vi "Timeout.vi"(8 "error in (no error)":errorcluster, 10 "allow send timeout":bool=TRUE, 11 "BaseDriver in":refnum<class "BaseDriver.lvclass">) -> (0 "error out":errorcluster, 2 "timed out?":bool, 3 "BaseDriver out":refnum<class "BaseDriver.lvclass">)   [LabVIEW 2013, in "BaseDriver.lvclass"]
doc: "Handles a timeout that occurs when an expected response to a message doesn't arrive on time. Tries to resend the message a fixed number of times"
uses:
  BaseDriver.lvclass
  BaseDriver.lvclass/BaseDriver.ctl
  Message/BaseMessage/BaseMessage.lvclass
  driver_state.ctl
  Responder/BaseResponder/BaseResponder.lvclass
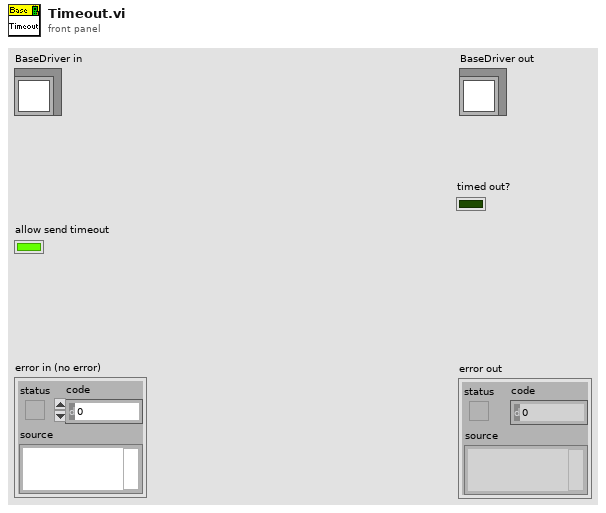
[diagram p1: front panel]
types:
  T1 = typedef "driver_state.ctl" = enum16{"Idle", "Wait for ack"}
  T2 = typedef "response.ctl" = cluster{"driver status":T3, "Sender":string, "Type":i32, "Variant":variant}
  T3 = typedef "driver_status.ctl" = enum16{"Normal", "Startup", "Connection lost", "Reconnected", "Timeout", "Idle", "Busy"}
  T4 = typedef "message_queue.ctl" = refnum<queue>
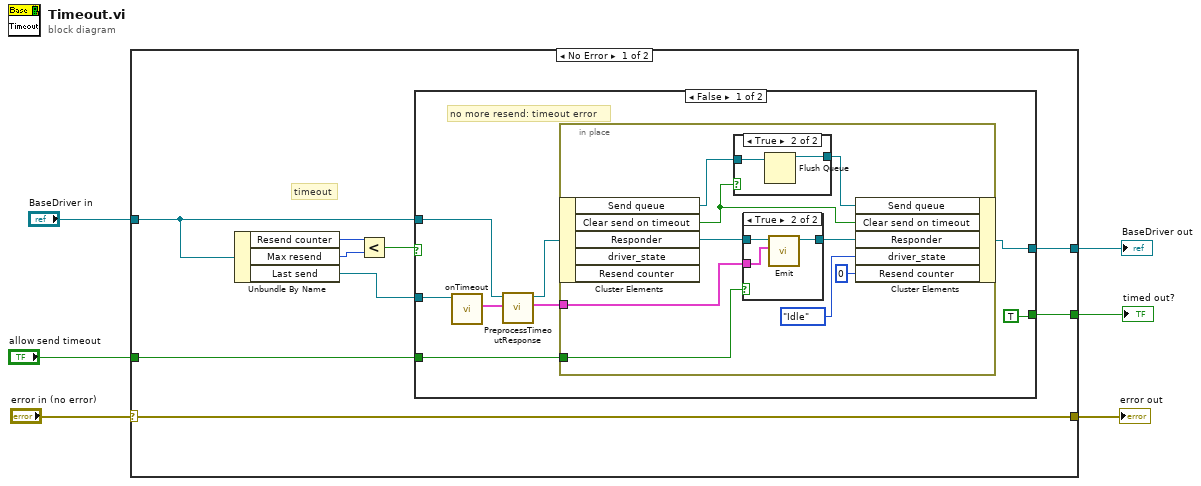
[diagram p0: block diagram]
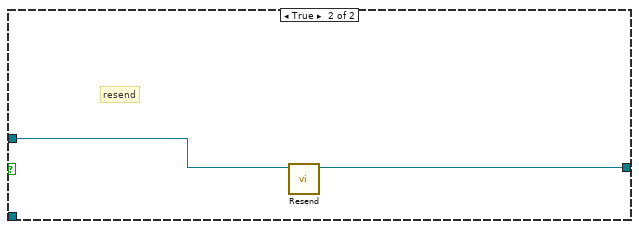
[diagram p4: hidden frame]
diagram:
  n1 = case shown="No Error" "error in (no error)" {
    selector: "error in (no error)" -> [w10 w42]
    tunnel: "BaseDriver in" -> [w12 w43]
    tunnel: [w11 w43] -> w5
    tunnel: [w10 w42] -> w3
    tunnel: [w8 _] -> w2
    tunnel: "allow send timeout" -> [w7 _]
    frame No Error {
      # "timeout"
      n2 = Unbundle By Name(w12) -> ("Resend counter"=w15:i32, "Max resend"=w14:i32, "Last send"=w9:refnum<class "BaseMessage.lvclass">)
      n3 = Less?(x=w15, y=w14) -> (x < y?=w13:bool)
      n4 = case shown="False" w13 {
        tunnel: w12 -> [w19 w41]
        tunnel: [w20 w40] -> w11
        tunnel: w9 -> [w23 _]
        tunnel: [TRUE _] -> w8
        tunnel: w7 -> [w21 _]
        frame False {
          # "no more resend: timeout error"
          n5 = call-dynamic "onTimeout.vi"("Last sent message in"=w23) -> ("response"=w17:T2)  [unwired: 8 in, 2 out]
          n6 = call-dynamic "PreprocessTimeoutResponse.vi"("response in"=w17, "BaseDriver In"=w19) -> ("response out"=w16:T2, "BaseDriver Out"=w18:refnum<class "BaseDriver.lvclass">)  [unwired: 7 in, 1 out]
          n7 = in-place "In Place Element Structure" {
            in-place-border: w16 -> [w32]
            in-place-border: w21 -> [w25]
            n8 = in-place-cluster #1(w18) -> ("Send queue"=w27:T4, "Clear send on timeout"=w24:bool, "Responder"=w31:refnum<class "BaseResponder.lvclass">)  [unwired: 2 out]
            n9 = case shown="True" w24 {
              tunnel: w27 -> [w37 w39]
              tunnel: [w37 w38] -> w26
              frame False {
              }
              frame True {
                n10 = Flush Queue(queue=w39) -> (queue out=w38:T4)  [unwired: 1 in, 2 out]
              }
            }
            n11 = case shown="True" w25 {
              tunnel: w32 -> [_ w36]
              tunnel: w31 -> [w33 w35]
              tunnel: [w33 w34] -> w30
              frame False {
              }
              frame True {
                n12 = call-dynamic "Emit.vi"("response"=w36, "BaseResponder in"=w35) -> ("BaseResponder out"=w34:refnum<class "BaseResponder.lvclass">)  [unwired: 8 in, 1 out]
              }
            }
            n13 = in-place-cluster #1("Send queue"=w26, "Clear send on timeout"=w24, "Responder"=w30, "driver_state"=driver_state."Idle", "Resend counter"=0) -> (w20:refnum<class "BaseDriver.lvclass">)
          }
        }
        frame True {
          # "resend"
          n14 = call "Resend.vi"("BaseDriver in"=w41) -> ("BaseDriver out"=w40:refnum<class "BaseDriver.lvclass">)  [unwired: 9 in, 1 out]
        }
      }
    }
    frame Error {
    }
  }
  "error out" <- w3
  "BaseDriver out" <- w5
  "timed out?" <- w2
